vi "CameraCOM.vi"() -> (0 "CamCOM":bool)   [LabVIEW 2011]
uses:
  Globals.vi
panel:
  in  "OK":bool
  out "Message":string="Le contrôleur de la caméra ne répond pas"
  in  "Retry":bool
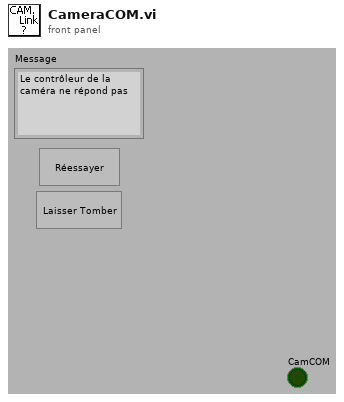
[diagram p1: front panel]
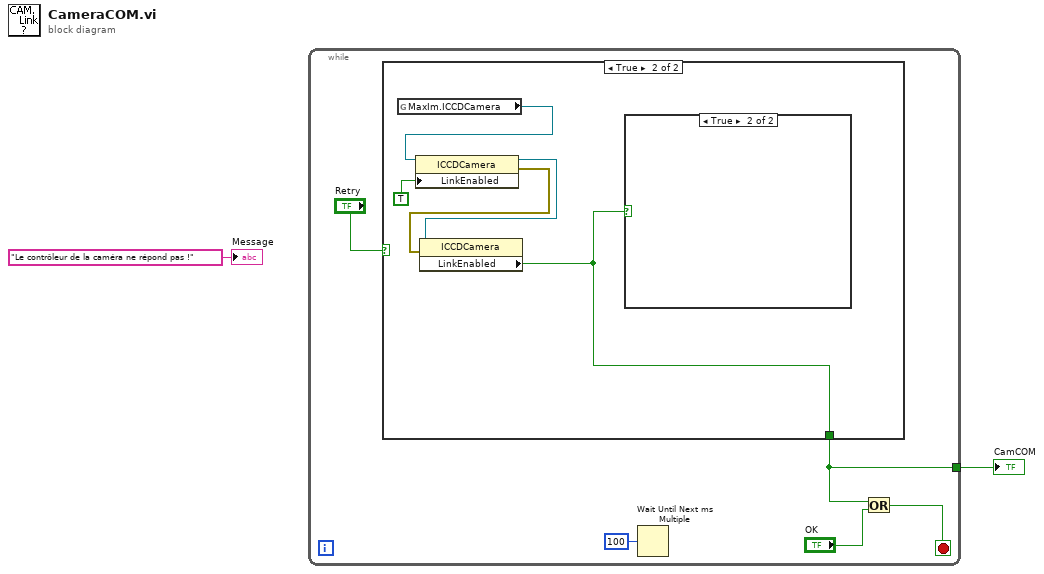
[diagram p0: block diagram]
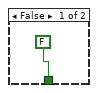
[diagram p2: hidden frame]
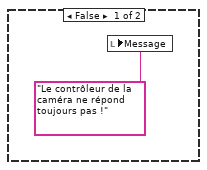
[diagram p3: hidden frame]
diagram:
  n1 = while {
    tunnel: [w4] -> w1
    stop <- w5 stop-if-true
    n2 = case shown="True" "Retry" {
      tunnel: [FALSE w12] -> w4
      frame False {
      }
      frame True {
        n3 = global read "Globals.vi" "MaxIm.ICCDCamera"() -> (w13:refnum<k7>)
        n4 = property class="ICCDCamera"(reference=w13, "LinkEnabled"=TRUE) -> (reference out=w11:refnum<k7>, error out=w10:errorcluster)  [unwired: 1 in]
        n5 = property class="ICCDCamera"(reference=w11, error in=w10) -> ("LinkEnabled"=w12:bool)  [unwired: 2 out]
        n6 = case shown="True" w12 {
          frame False {
            n7 = local write "Message"("Le contrôleur de la caméra ne répond toujours pas !" ("Message")) -> ()
          }
          frame True {
          }
        }
      }
    }
    n8 = Wait Until Next ms Multiple(millisecond multiple=u32 100 ("n millisecondes")) -> ()  [unwired: 1 out]
    n9 = Or(x=w4, y="OK") -> (x .or. y?=w5:bool)
  }
  "CamCOM" <- w1
  "Message" <- "Le contrôleur de la caméra ne répond pas !" ("Message")
